vi "Program_3_three_filtered_sine_waves.vi"() -> ()   [LabVIEW 2015]
uses:
  <vilib>/measure/NI_MABase.lvlib
panel:
  out "Waveform Graph 7":waveform(dbl)(graph)={"t0"=timestamp(0 s since 1904-01-01), "dt"=0.01, "Y"=[0.0, 0.3090169943749474, 0.587785252292473, 0.8090169943749473, 0.9510565162951534, 1.0, 0.9510565162951535, 0.8090169943749476, 0.5877852522924732, 0.30901699437494773, 2.220446049250313e-16, -0.30901699437494706, -0.5877852522924728, -0.8090169943749472, -0.9510565162951534, -1.0, -0.9510565162951536, -0.8090169943749477, -0.5877852522924734, -0.30901699437494795, -3.3306690738754696e-16, 0.30901699437494673, 0.5877852522924728, 0.809016994374947, 0.9510565162951534, 1.0, 0.9510565162951536, 0.8090169943749479, 0.5877852522924734, 0.3090169943749482, 3.3306690738754696e-16, -0.3090169943749466, -0.5877852522924728, -0.8090169943749468, -0.9510565162951534, -0.9999999999999999, -0.9510565162951536, -0.809016994374948, -0.5877852522924734, -0.3090169943749485, -3.3306690738754696e-16, 0.3090169943749462, 0.5877852522924728, 0.8090169943749466, 0.9510565162951534, 0.9999999999999999, 0.9510565162951536, 0.8090169943749482, 0.5877852522924734, 0.3090169943749489, 3.3306690738754696e-16, -0.3090169943749458, -0.5877852522924728, -0.8090169943749463, -0.9510565162951534, -0.9999999999999999, -0.9510565162951536, -0.8090169943749485, -0.5877852522924734, -0.3090169943749493, -3.3306690738754696e-16, 0.3090169943749454, 0.5877852522924728, 0.8090169943749459, 0.9510565162951534, 0.9999999999999997, 0.9510565162951536, 0.8090169943749486, 0.5877852522924734, 0.3090169943749496, 3.3306690738754696e-16, -0.30901699437494495, -0.5877852522924728, -0.8090169943749457, -0.9510565162951534, -0.9999999999999997, -0.9510565162951536, -0.8090169943749488, -0.5877852522924734, -0.30901699437495, -3.3306690738754696e-16, 0.3090169943749447, 0.5877852522924728, 0.8090169943749456, 0.9510565162951534, 0.9999999999999998, 0.9510565162951536, 0.809016994374949, 0.5877852522924734, 0.3090169943749503, 3.3306690738754696e-16, -0.3090169943749444, -0.5877852522924728, -0.8090169943749455, -0.9510565162951534, -0.9999999999999998, -0.9510565162951536, -0.8090169943749492, -0.5877852522924734, -0.3090169943749505]}
  out "Waveform Graph 6":waveform(dbl)(graph)={"t0"=timestamp(0 s since 1904-01-01), "dt"=0.01, "Y"=[0.0, 0.12533323356430426, 0.24868988716485482, 0.368124552684678, 0.4817536741017153, 0.5877852522924731, 0.6845471059286887, 0.7705132427757893, 0.8443279255020152, 0.9048270524660196, 0.9510565162951536, 0.9822872507286887, 0.9980267284282717, 0.9980267284282716, 0.9822872507286887, 0.9510565162951535, 0.9048270524660196, 0.844327925502015, 0.7705132427757893, 0.6845471059286885, 0.5877852522924731, 0.481753674101715, 0.3681245526846779, 0.24868988716485443, 0.12533323356430418, -3.885780586188048e-16, -0.12533323356430434, -0.24868988716485518, -0.36812455268467803, -0.48175367410171566, -0.5877852522924731, -0.684547105928689, -0.7705132427757893, -0.8443279255020153, -0.9048270524660196, -0.9510565162951536, -0.9822872507286887, -0.9980267284282716, -0.9980267284282716, -0.9822872507286885, -0.9510565162951535, -0.9048270524660192, -0.844327925502015, -0.7705132427757888, -0.6845471059286885, -0.5877852522924726, -0.481753674101715, -0.36812455268467736, -0.24868988716485443, -0.12533323356430362, 3.885780586188048e-16, 0.12533323356430484, 0.24868988716485518, 0.3681245526846785, 0.48175367410171566, 0.5877852522924736, 0.684547105928689, 0.7705132427757895, 0.8443279255020153, 0.9048270524660196, 0.9510565162951536, 0.9822872507286886, 0.9980267284282716, 0.9980267284282713, 0.9822872507286885, 0.9510565162951532, 0.9048270524660192, 0.8443279255020145, 0.7705132427757888, 0.684547105928688, 0.5877852522924726, 0.48175367410171444, 0.36812455268467736, 0.24868988716485385, 0.12533323356430362, -9.71445146547012e-16, -0.12533323356430484, -0.24868988716485574, -0.3681245526846785, -0.48175367410171616, -0.5877852522924736, -0.6845471059286894, -0.7705132427757895, -0.8443279255020156, -0.9048270524660196, -0.9510565162951539, -0.9822872507286886, -0.9980267284282716, -0.9980267284282713, -0.9822872507286884, -0.9510565162951532, -0.9048270524660189, -0.8443279255020145, -0.7705132427757884, -0.684547105928688, -0.587785252292472, -0.48175367410171444, -0.3681245526846767, -0.24868988716485385, -0.12533323356430293]}
  out "Waveform Graph 5":waveform(dbl)(graph)={"t0"=timestamp(0 s since 1904-01-01), "dt"=0.01, "Y"=[0.0, 0.5877852522924731, 0.9510565162951536, 0.9510565162951536, 0.5877852522924731, 0.0, -0.5877852522924731, -0.9510565162951536, -0.9510565162951536, -0.5877852522924731, 0.0, 0.5877852522924731, 0.9510565162951536, 0.9510565162951536, 0.5877852522924731, 0.0, -0.5877852522924731, -0.9510565162951536, -0.9510565162951536, -0.5877852522924731, 0.0, 0.5877852522924731, 0.9510565162951536, 0.9510565162951536, 0.5877852522924731, 0.0, -0.5877852522924731, -0.9510565162951536, -0.9510565162951536, -0.5877852522924731, 0.0, 0.5877852522924731, 0.9510565162951536, 0.9510565162951536, 0.5877852522924731, 0.0, -0.5877852522924731, -0.9510565162951536, -0.9510565162951536, -0.5877852522924731, 0.0, 0.5877852522924731, 0.9510565162951536, 0.9510565162951536, 0.5877852522924731, 0.0, -0.5877852522924731, -0.9510565162951536, -0.9510565162951536, -0.5877852522924731, 0.0, 0.5877852522924731, 0.9510565162951536, 0.9510565162951536, 0.5877852522924731, 0.0, -0.5877852522924731, -0.9510565162951536, -0.9510565162951536, -0.5877852522924731, 0.0, 0.5877852522924731, 0.9510565162951536, 0.9510565162951536, 0.5877852522924731, 0.0, -0.5877852522924731, -0.9510565162951536, -0.9510565162951536, -0.5877852522924731, 0.0, 0.5877852522924731, 0.9510565162951536, 0.9510565162951536, 0.5877852522924731, 0.0, -0.5877852522924731, -0.9510565162951536, -0.9510565162951536, -0.5877852522924731, 0.0, 0.5877852522924731, 0.9510565162951536, 0.9510565162951536, 0.5877852522924731, 0.0, -0.5877852522924731, -0.9510565162951536, -0.9510565162951536, -0.5877852522924731, 0.0, 0.5877852522924731, 0.9510565162951536, 0.9510565162951536, 0.5877852522924731, 0.0, -0.5877852522924731, -0.9510565162951536]}
  out "Waveform Graph 4":dynamicdata(graph)=[{"t0"=timestamp(0 s since 1904-01-01), "dt"=0.01, "Y"=[0.0, 0.003701849174507947, 0.019958918872853837, 0.0539596390806561, 0.10055767031208249, 0.14607423938727265, 0.17337149158685822, 0.1682448506692858, 0.12475223278120182, 0.047557455852924035, -0.04947342673161903, -0.1477699502549087, -0.2298675604853475, -0.28432785364114643, -0.3079998453521582, -0.3049591966001346, -0.28280098700667855, -0.24800757679697916, -0.20245754820654804, -0.14265032477668893, -0.06208583161331138, 0.04409597245823843, 0.17411880439545857, 0.3163972826133177, 0.44978880689209666, 0.5476396032759766, 0.5845680331517724, 0.5438456839972561, 0.42291280169046463, 0.23513187113120293, 0.007140403738758461, -0.22734865809531857, -0.43527840965199227, -0.5910592014547175, -0.680461784450529, -0.7007472642633958, -0.6575927854998211, -0.5604923345889656, -0.41873049290143816, -0.239600263070328, -0.029449290211562285, 0.2031679718417886, 0.44395705914577177, 0.6709869602796452, 0.8559019977277522, 0.9685277038738547, 0.9837812754558084, 0.888765560592371, 0.6876462355406616, 0.40251286187494584, 0.06970176087989244, -0.26744886967075576, -0.5672780489774474, -0.7973709494046745, -0.9389567787787463, -0.9872608760039041, -0.9483738938686233, -0.8343512848776133, -0.6586979219153872, -0.4339804991137184, -0.17222866207090037, 0.11252488134302618, 0.40122905665638586, 0.6682976186304297, 0.8830387250930872, 1.014313120604185, 1.0373467307416608, 0.9406065336294986, 0.73037886684667, 0.4312943282477115, 0.08231921536900977, -0.27078014557965524, -0.5843401581846666, -0.8245102707976021, -0.9717064089448433, -1.020939769381482, -0.9785991286830535, -0.8574205251905678, -0.6718219319231831, -0.4353674132022225, -0.1610400405321144, 0.13631320110541978, 0.4370216014306577, 0.7150893014961927, 0.9396052582786814, 1.0793560748104603, 1.1095790986154435, 1.0187767406500883, 0.8132420155306193, 0.5175476872420695, 0.17052369300871462, -0.1822698963425693, -0.49741704795017605, -0.7413131432175348, -0.8945686172107105, -0.9522893073059955, -0.9208193798723534, -0.8126868858522349], "attributes"=variant("NI_ChannelName"=variant(string "Filtered"))}]
  out "Waveform Graph 3":dynamicdata(graph)=[{"t0"=timestamp(0 s since 1904-01-01), "dt"=0.01, "Y"=[0.0, 1.3587991971997144e-05, 0.00012738884622537456, 0.0005990301419269113, 0.0019155324068872161, 0.004747297674294699, 0.009808496590156543, 0.01767989695383657, 0.028656566853590467, 0.04266771194912412, 0.059285522525306875, 0.07780613524137822, 0.09736142509024064, 0.11701419533951031, 0.13580305146777621, 0.15273067857501602, 0.16671891259599986, 0.1765735890934667, 0.1810033244144903, 0.178718034407091, 0.16860176151558415, 0.14992213604173799, 0.1225181253801928, 0.08690708676726855, 0.04427258428184677, -0.0036708831845677636, -0.054903387893882716, -0.10735675792534938, -0.15913915891515806, -0.2086786007879322, -0.25476786900840587, -0.29652767371117417, -0.3333296458783632, -0.3647273191322986, -0.3904297903853484, -0.41032550309854265, -0.42453402431101406, -0.4334441119209895, -0.4376951456769831, -0.4380772327826685, -0.4353563731620449, -0.4300631189747097, -0.42230361730779187, -0.41165233628730746, -0.39716510550927797, -0.3775162053768626, -0.35122634456506674, -0.31692250888313567, -0.2735648197364301, -0.22059127233212017, -0.1579621608446269, -0.08612030012769267, -0.00590803920112748, 0.08151134117961245, 0.17469357920002437, 0.27190756503761904, 0.37110589517661907, 0.4699134810208587, 0.5656768823091518, 0.6555986154802227, 0.7369494400626984, 0.8073194204578229, 0.864847972740435, 0.90837258917405, 0.9374565285855709, 0.9522906176166828, 0.9535011997256255, 0.9419221574205743, 0.9183948461058442, 0.8836441468572538, 0.8382480391286293, 0.7826839485935722, 0.7174104172719638, 0.6429362392436211, 0.559842733025242, 0.4687521305925646, 0.3702646729335566, 0.26490659358497837, 0.15313239335768358, 0.03540655531828474, -0.08764125413172297, -0.21502554006723384, -0.3452374303527952, -0.47615922259168375, -0.6050994037771158, -0.728951668222118, -0.8444446042399392, -0.9484228981375722, -1.0380950856815119, -1.111198631769252, -1.1660640665488344, -1.201594211146375, -1.2171994071843422, -1.2127362506571409, -1.1884839906985967, -1.1451656334781717, -1.0839913668287515, -1.0066825075968282], "attributes"=variant("NI_ChannelName"=variant(string "Filtered"))}]
  out "Waveform Graph 2":dynamicdata(graph)=[{"t0"=timestamp(0 s since 1904-01-01), "dt"=0.01, "Y"=[0.0, 0.4031068755426856, -0.030093805902072, -0.4679846947208353, -0.5442718366177486, -0.25062169984105, 0.21022084293026086, 0.5805130331896872, 0.6758662207046815, 0.45605656988408616, 0.026522093020620252, -0.4190305470720982, -0.6862651016016106, -0.6617060238575394, -0.35695126706911906, 0.09948162913337488, 0.5170712181426931, 0.7217017987061218, 0.6260705089008904, 0.2645791341738368, -0.2204242096335483, -0.635085571358815, -0.8107175731508436, -0.6706328293658834, -0.26110601251921284, 0.26553799302591524, 0.7091510931885048, 0.8987991840057559, 0.7588749949691511, 0.33877553162349505, -0.20534694200611037, -0.669834844975719, -0.8811053814991967, -0.7618466260382175, -0.36046371491001805, 0.16752396042276874, 0.6190389616989017, 0.8211797489094621, 0.6973915704688542, 0.29674780023458514, -0.2248794925366625, -0.6645789185492562, -0.8502464153471867, -0.7067442071988177, -0.2850469659892445, 0.25681592921968044, 0.713794564887082, 0.9119364057315495, 0.774770336465803, 0.3526029153400576, -0.1964772411600484, -0.6666582226882, -0.882622243051558, -0.7660859961577682, -0.36528933946050524, 0.16379243658179488, 0.617303165928953, 0.8215396167676166, 0.6993432368021038, 0.2994867893747759, -0.2221606324153057, -0.6624764170150798, -0.8490479891842013, -0.7064414183234646, -0.2854227488802954, 0.2560693254154488, 0.7129673759060968, 0.9112290312769535, 0.7742660192700663, 0.3522799220141075, -0.19670843210716693, -0.666909788656247, -0.8829902844696922, -0.7666267676999121, -0.36601258488876587, 0.16291607831172916, 0.6163266088925622, 0.8205220454146058, 0.698336144771188, 0.29852606810780213, -0.22305621854192093, -0.6633018334726578, -0.8498059737589438, -0.7071363356849716, -0.2860560027339363, 0.25550149296443325, 0.712473746137813, 0.9108215964360955, 0.7739574248154706, 0.35208103394434254, -0.19679023841554266, -0.6668713768277474, -0.8828326199907579, -0.7663541798643307, -0.3656317848959918, 0.16339690936804452, 0.61689846295144, 0.821175396915691], "attributes"=variant("NI_ChannelName"=variant(string "Filtered"))}]
  out "Waveform Graph":waveform(dbl)(graph)={"t0"=timestamp(0 s since 1904-01-01), "dt"=0.01, "Y"=[0.0, 1.0221354802317248, 1.7875316557524816, 2.128198063354779, 2.020595442689342, 1.5877852522924731, 1.047818369931369, 0.6284737208555832, 0.4810566614993348, 0.6260587945484941, 0.9510565162951539, 1.2610555086462147, 1.3612979924309525, 1.140066250348478, 0.6190159867260083, -0.04894348370484647, -0.6340147161216072, -0.9157455851680864, -0.7683285258118377, -0.21225514073873258, 0.5877852522924728, 1.378555920769135, 1.9069663212723045, 2.0087633978349553, 1.6641750021519308, 0.9999999999999996, 0.23793803043837614, -0.3907294090850608, -0.7313958166873582, -0.7605219320192407, -0.5877852522924728, -0.40577884801116243, -0.4072419787731084, -0.7022884035818084, -1.2680983164686999, -1.9510565162951536, -2.5211290193163154, -2.7581002390983733, -2.536868497015899, -1.8790894973961103, -0.9510565162951539, -0.008024805798599932, 0.6945138430856115, 0.9895602678943114, 0.854294662658938, 0.4122147477075273, -0.11848241009903449, -0.5101640746048829, -0.6119611511675347, -0.40410149148182783, 7.216449660063518e-16, 0.40410149148183216, 0.6119611511675359, 0.5101640746048857, 0.11848241009903537, -0.4122147477075263, -0.8542946626589378, -0.9895602678943126, -0.6945138430856117, 0.008024805798597157, 0.9510565162951533, 1.8790894973961072, 2.536868497015898, 2.758100239098371, 2.521129019316315, 1.9510565162951528, 1.2680983164686999, 0.7022884035818094, 0.4072419787731085, 0.40577884801116443, 0.5877852522924729, 0.7605219320192427, 0.7313958166873583, 0.3907294090850617, -0.2379380304383767, -1.0000000000000007, -1.6641750021519317, -2.008763397834958, -1.9069663212723054, -1.3785559207691391, -0.5877852522924739, 0.21225514073872842, 0.768328525811837, 0.9157455851680836, 0.634014716121607, 0.048943483704845914, -0.6190159867260081, -1.1400662503484762, -1.3612979924309516, -1.2610555086462112, -0.9510565162951529, -0.6260587945484901, -0.4810566614993337, -0.6284737208555802, -1.0478183699313681, -1.5877852522924718, -2.0205954426893413, -2.1281980633547795]}
  in  "sampling info 3":cluster{"Fs":dbl, "#s":dbl}={"Fs"=100.0, "#s"=100.0} {"Fs" format="%.2p"}
  in  "phase 3":dbl format="%.2p"
  in  "amplitude 3":dbl=1.0 format="%0.2p"
  in  "frequency 3":dbl=5.0 format="%0.2p"
  in  "sampling info 2":cluster{"Fs":dbl, "#s":dbl}={"Fs"=100.0, "#s"=100.0} {"Fs" format="%.2p"}
  in  "phase 2":dbl format="%.2p"
  in  "amplitude 2":dbl=1.0 format="%0.2p"
  in  "frequency 2":dbl=2.0 format="%0.2p"
  in  "sampling info":cluster{"Fs":dbl, "#s":dbl}={"Fs"=100.0, "#s"=98.0} {"Fs" format="%.2p"}
  in  "phase":dbl format="%.2p"
  in  "amplitude":dbl=1.0 format="%0.2p"
  in  "frequency":dbl=10.0 format="%0.2p"
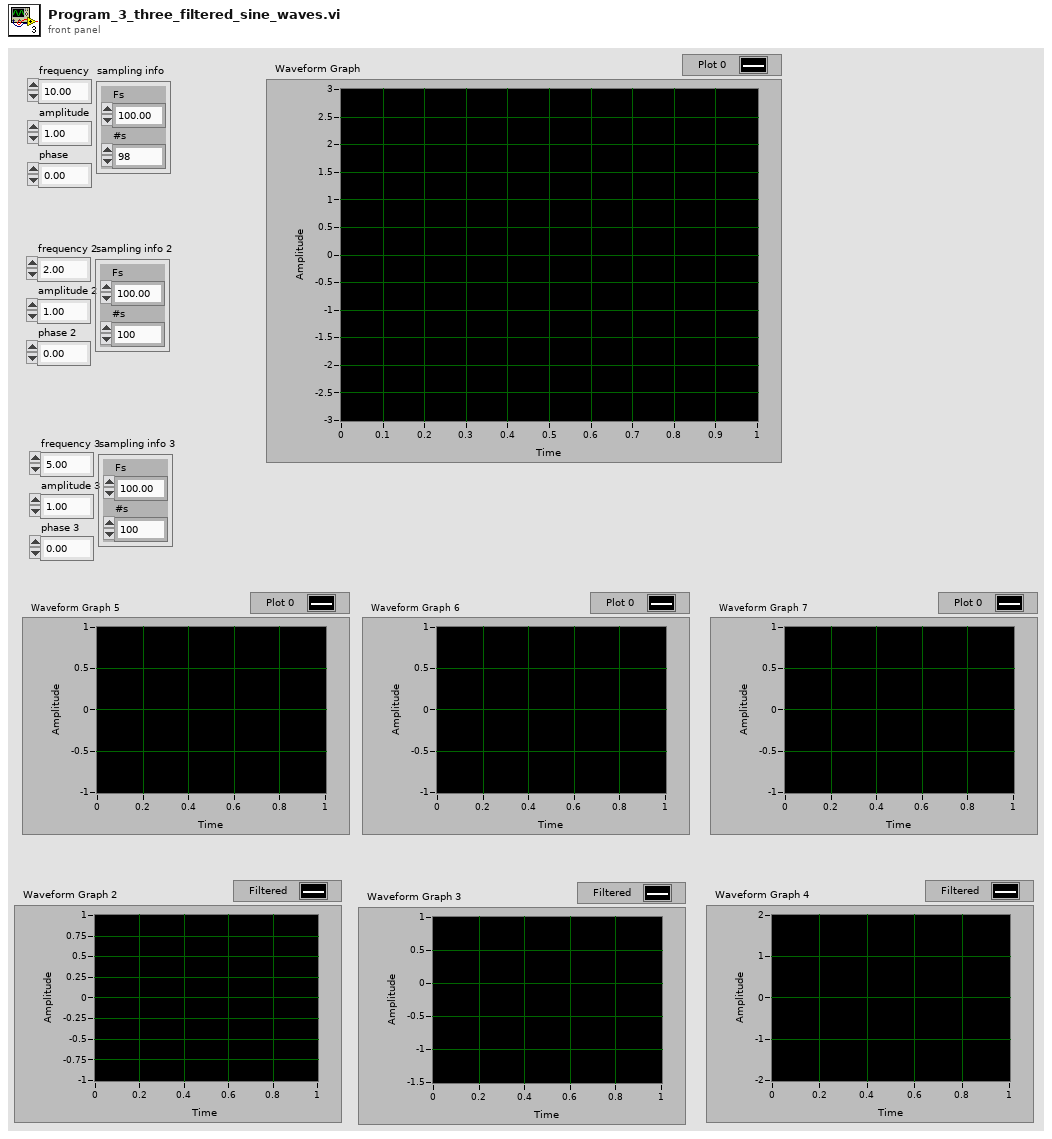
[diagram p1: front panel]
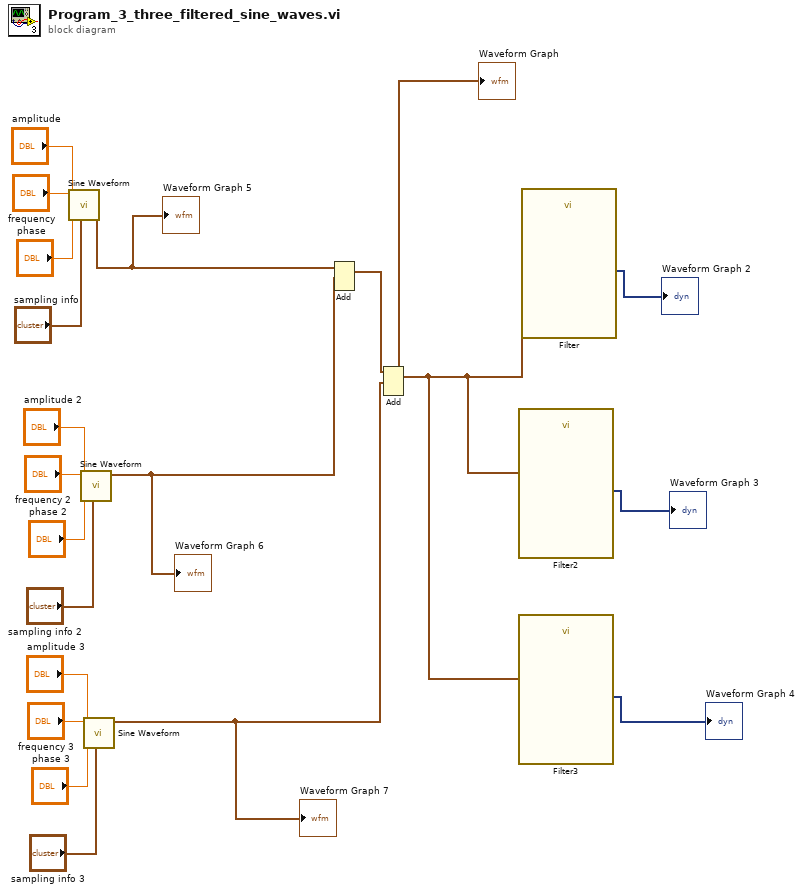
[diagram p0: block diagram]
diagram:
  n1 = call <vilib>:"Sine Waveform.vi"("sampling info"="sampling info", "phase"="phase", "amplitude"="amplitude", "frequency"="frequency") -> ("signal out"=w3:waveform(dbl))  [unwired: 6 in, 1 out]
  "Waveform Graph 5" <- w3
  n2 = call <vilib>:"Sine Waveform.vi"("sampling info"="sampling info 2", "phase"="phase 2", "amplitude"="amplitude 2", "frequency"="frequency 2") -> ("signal out"=w2:waveform(dbl))  [unwired: 6 in, 1 out]
  "Waveform Graph 6" <- w2
  n3 = call <vilib>:"Sine Waveform.vi"("sampling info"="sampling info 3", "phase"="phase 3", "amplitude"="amplitude 3", "frequency"="frequency 3") -> ("signal out"=w1:waveform(dbl))  [unwired: 6 in, 1 out]
  "Waveform Graph 7" <- w1
  n4 = Add(1:w2, 2:w3) -> (0:w8:waveform(dbl))  [unwired: 1 in, 1 out]
  n5 = Add(1:w1, 2:w8) -> (0:w7:waveform(dbl))  [unwired: 1 in, 1 out]
  "Waveform Graph" <- w7
  n6 = call "Filter2"("Signal"=w7) -> ("Filtered Signal"=→"Waveform Graph 3":dynamicdata)  [unwired: 9 in, 1 out]
  n7 = call "Filter3"("Signal"=w7) -> ("Filtered Signal"=→"Waveform Graph 4":dynamicdata)  [unwired: 9 in, 1 out]
  n8 = call "Filter"("Signal"=w7) -> ("Filtered Signal"=→"Waveform Graph 2":dynamicdata)  [unwired: 9 in, 1 out]
